vi "SubVI_CaptureIR.vi"(0 "ErrorIn":errorcluster, 1 "af1DTempMat":sgl[](array[numeric]), 2 "u8PaletteType":u8, 5 "au8Channel-B":u8[](array[numeric]), 9 "au8Channel-G":u8[](array[numeric]), 11 "au8Channel-R":u8[](array[numeric])) -> (3 "af2DTempMat":sgl[][](array[numeric]), 4 "ErrorOut":errorcluster caption="ErrorOut)", 6 "au8Channel-B":u8[](array[numeric]), 10 "au8Channel-G":u8[](array[numeric]), 12 "i32Width":i32, 13 "i32Height":i32, 14 "u8Error":u8, 15 "au8Channel-R":u8[](array[numeric]))   [LabVIEW 2013]
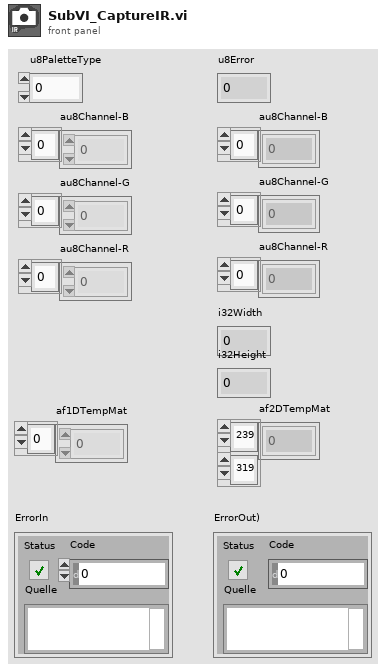
[diagram p1: front panel]
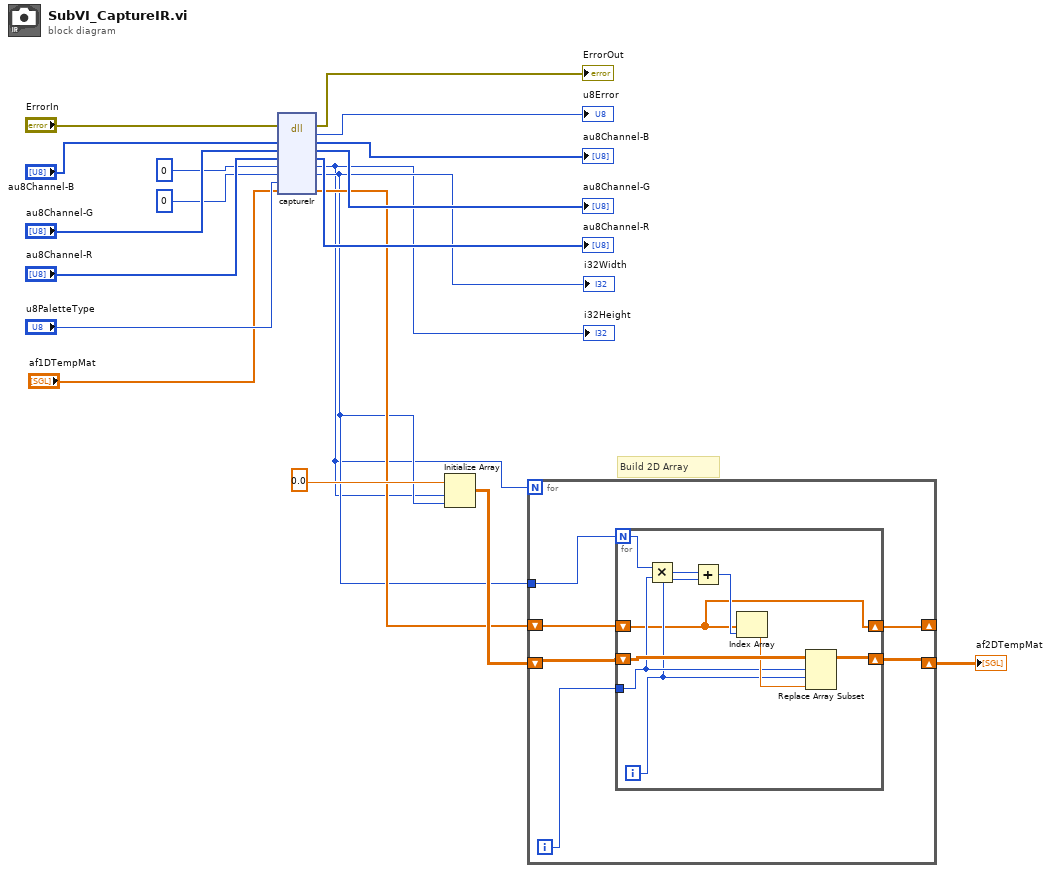
[diagram p0: block diagram]
diagram:
  # "Build 2D Array"
  n1 = dll-call lib="PTH1abs CUsers1000len-bimDesktop&Lieferung_LabView_Interface_11.11.2015Einrichten fÃ¼r - EndkundenDatenTesto_v2013VIlabview_cwrapper_1_0_0.dll" fn="captureIr"(error in="ErrorIn", "au8ChannelB"="au8Channel-B", "au8ChannelG"="au8Channel-G", "au8ChannelR"="au8Channel-R", "i32Height"=0, "i32Width"=0, "u8PaletteType"="u8PaletteType", "af2DTempMat"="af1DTempMat") -> (error out=→"ErrorOut":errorcluster, "u8Error"=→"u8Error":u8, "au8ChannelB"=→"au8Channel-B":u8[], "au8ChannelG"=→"au8Channel-G":u8[], "au8ChannelR"=→"au8Channel-R":u8[], "i32Height"=w1:i32, "i32Width"=w2:i32, "af2DTempMat"=w3:sgl[])  [unwired: 3 in, 1 out]
  "i32Width" <- w2
  "i32Height" <- w1
  n2 = Initialize Array(sgl 0.0 ("Element"), w1, w2) -> (w5:sgl[][])
  n3 = for {
    N: w1 -> [_]
    shift-right: [w24] -> w4
    shift-left: w5 -> [w25]
    tunnel: w2 -> [w22]
    shift-right: [w20] -> _
    shift-left: w3 -> [w21]
    i -> [w23]
    n4 = for {
      N: w22 -> [w31]
      shift-right: [w33] -> w24
      shift-left: w25 -> [w34]
      tunnel: w23 -> [w30]
      shift-right: [w26] -> w20
      shift-left: w21 -> [w26]
      i -> [w28]
      n5 = Multiply(x=w31, y=w30) -> (x*y=w29:i32)
      n6 = Add(x=w29, y=w28) -> (x+y=w27:i32)
      n7 = Index Array(array=w26, index=w27) -> (element=w32:sgl)
      n8 = Replace Array Subset(array=w34, new element=w32, index (row)=w30, index (col)=w28) -> (w33:sgl[][])
    }
  }
  "af2DTempMat" <- w4
